vi "Set Z Acceleration.vi"(8 "error in (no error)":errorcluster, 10 "mm/s":dbl=15.0 format="%#_13g", 11 "Gantry In":refnum<k24>) -> (0 "error out":errorcluster, 3 "Gantry Out":refnum<k24>)   [LabVIEW 2018, in "A3200.lvclass"]
uses:
  A3200.lvclass
  C:/Program Files (x86)/Aerotech/A3200/LabVIEW/2010/Bin/Aerotech.A3200.dll
  Program Files (x86)/Aerotech/A3200/LabVIEW/2010/Bin/Aerotech.A3200.dll
  Drivers/Aerotech A3200/Aerotech.lvlib
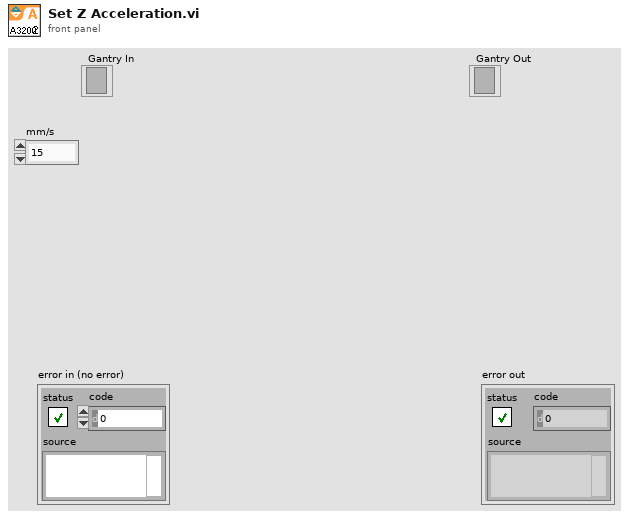
[diagram p1: front panel]
types:
  T1 = cluster{"Status":bool, "Error Code":i32, "Source":string}
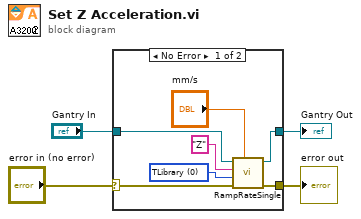
[diagram p0: block diagram]
diagram:
  n1 = case shown="No Error" "error in (no error)" {
    selector: "error in (no error)" -> [w5 w12]
    tunnel: "Gantry In" -> [w11 w13]
    tunnel: [w10 w13] -> w3
    tunnel: [w9 w12] -> w2
    frame No Error {
      w6 = 0 items=["TLibrary", "T01", "T02", "T03", "T04", "T05", "T06", "T07", "T08", "T09", "T10", "T11", "T12", "T13", "T14", "T15", "T16", "T17", "T18", "T19", "T20", "T21", "T22", "T23", "T24", "T25", "T26", "T27", "T28", "T29", "T30", "T31"] ("task id")
      n2 = call "RampRateSingle.vi"("ramp rate"="mm/s", "error in (no error)"=w5, "task id"=w6, "axis name"="Z", "controller in"=w11) -> ("error out (no error)"=w9:T1, "controller out"=w10:refnum<k24>)  [unwired: 5 in]
    }
    frame Error {
    }
  }
  "error out" <- w2
  "Gantry Out" <- w3
